vi "Synth Cfg to Program.vi"(6 "Match clocks":bool, 7 "Mode":T2(ring), 8 "Clock Multiplier":u32=64, 9 "IF (Hz)":dbl, 10 "f (Hz)":dbl=100.0, 11 "Phase (degrees)":dbl=90.0) -> (0 "IF":u32, 1 "f":u32, 2 "Full Byte Array":u8[](array[numeric]) format="%08b", 3 "Clock F-word":u32, 4 "Fixed F-word":u32, 5 "Actual ratios":T1 {"Clock" format="%_20p"; "F2" format="%_20p"; "F1" format="%_20p"; "Clock/F2" format="%_20g"; "Clock/F1" format="%_20g"})   [LabVIEW 2016]
uses:
  Actual Settings.ctl
panel:
  # "33"
  # "65"
  # "1"
  # "40"
  # "72"
  # "8"
  # "Mode"
  # "function          J7          P3\n              syn1 w clk       A0           3\n              syn1 D7           A1           5\n              syn2 w clk       A2           7\n              syn2 D7           A3           9\n              syn3 w clk       A4           4\n              syn3 D7           A5           6\n              syn1,2 FQ_UD  A6           8\n              syn3 FQ_UD     A7          10\n\n              Reset 1,2,3     B4          14\n\n              SCLK              B0           13\n              SYNC              B1           15\n              DIN                B2           17"
  # "48"
  # "80"
  # "16"
  # "56"
  # "88"
  # "24"
  # "64"
  # "96"
  # "32"
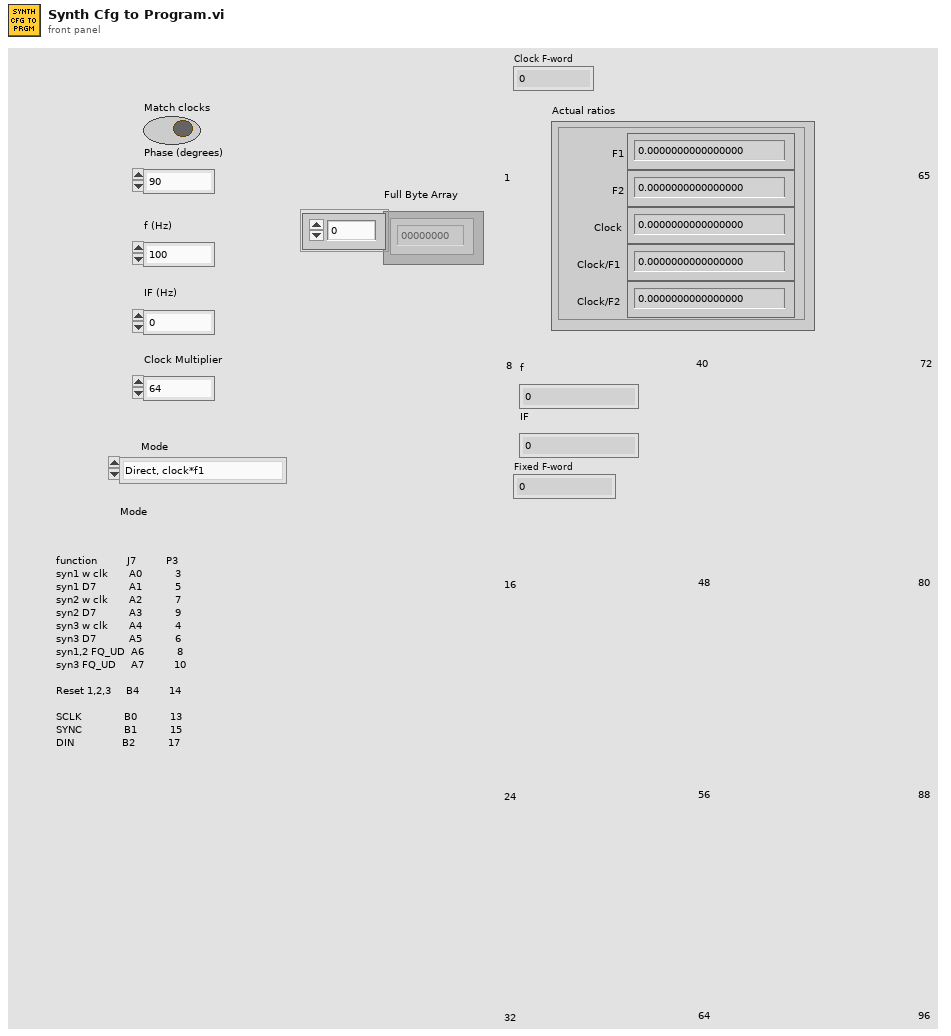
[diagram p1: front panel]
types:
  T1 = typedef "Actual settings.ctl" = cluster{"Clock/F1":ext, "Clock/F2":ext, "F1":ext, "F2":ext, "Clock":ext}
  T2 = enum16{"Direct, clock*f1", "Direct, clock*f2", "Heterodyne"}
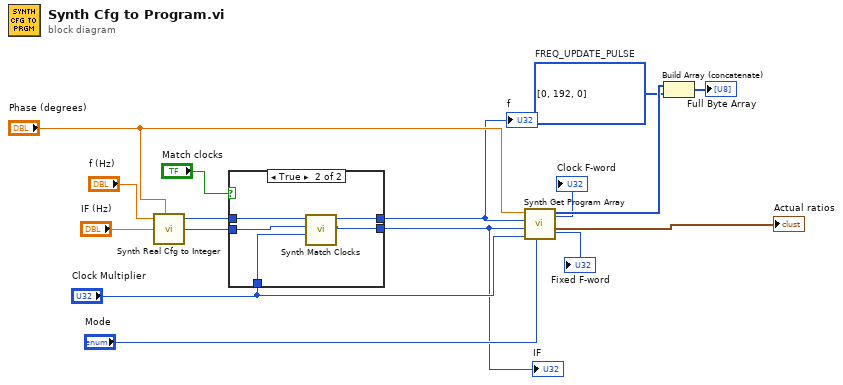
[diagram p0: block diagram]
diagram:
  w11 = u8[] [0, 192, 0]  # FREQ_UPDATE_PULSE
  n1 = call "Synth Real Cfg to Integer.vi"("Frequency(kHz)"="f (Hz)", "Phase(Degrees)"="Phase (degrees)", "IF (Hz)"="IF (Hz)") -> ("f-word"=w8:u32, "IF"=w7:u32)  [unwired: 4 in, 1 out]
  n2 = case shown="True" "Match clocks" {
    tunnel: w8 -> [w18 w23]
    tunnel: w7 -> [w17 w22]
    tunnel: "Clock Multiplier" -> [_ w21]
    tunnel: [w18 w20] -> w4
    tunnel: [w17 w19] -> w3
    frame False {
    }
    frame True {
      n3 = call "Synth Match Clocks.vi"("F1 Clock mutiplier"=w21, "F2"=w22, "F1"=w23) -> ("New F2"=w19:u32, "New F1"=w20:u32)  [unwired: 4 in, 3 out]
    }
  }
  "f" <- w4
  "IF" <- w3
  n4 = call "Synth Get Program Array.vi"("Mode"="Mode", "Clock multiplier"="Clock Multiplier", "Local Oscillator (IF,f2)"=w3, "f (f1)"=w4, "Phase (degrees)"="Phase (degrees)") -> ("Actual ratios"=→"Actual ratios":T1, "output array"=w13:u8[], "Fixed F-word"=→"Fixed F-word":u32, "Clock F-word"=→"Clock F-word":u32)  [unwired: 3 in]
  n5 = Build Array (concatenate)(w13, w11) -> (→"Full Byte Array":u8[])
